vi "relay ladder.vi"() -> ()   [LabVIEW 2013]
panel:
  out "Array 2":bool[](array[boolean])
  in  "Knob 2":i32(knob) scale=0.0..250.0
  in  "stop 2":bool
  in  "Knob":i32(knob) scale=0.0..250.0
  in  "stop":bool
  out "Array":bool[](array[boolean])
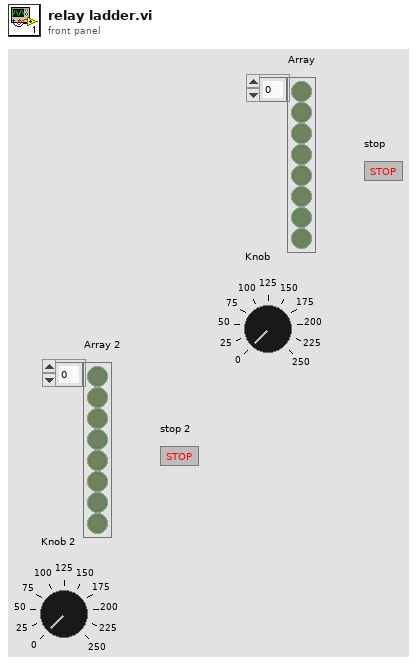
[diagram p1: front panel]
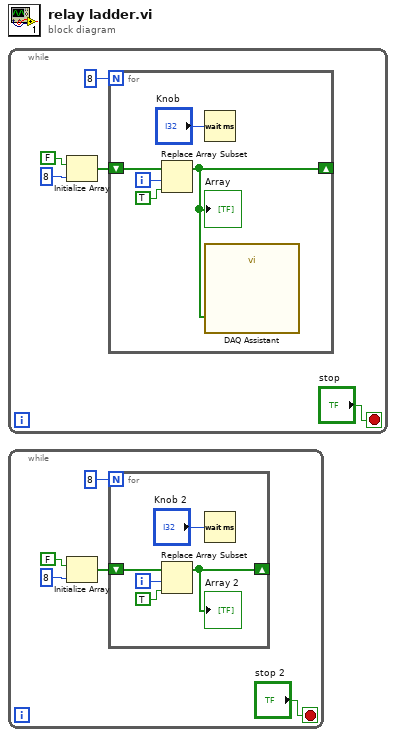
[diagram p0: block diagram]
diagram:
  n1 = while {
    stop <- "stop" stop-if-true
    n2 = Initialize Array(FALSE, 8 ("dimension size")) -> (w5:bool[])
    n3 = for {
      N: 8 -> [_]
      shift-right: [w7] -> _
      shift-left: w5 -> [w10]
      i -> [w9]
      n4 = Replace Array Subset(array=w10, new element=TRUE, index=w9) -> (w7:bool[])
      "Array" <- w7
      n5 = Wait (ms)(milliseconds to wait="Knob") -> ()  [unwired: 1 out]
      n6 = call "DAQ Assistant"("data"=w7) -> ()  [unwired: 17 in, 2 out]
    }
  }
  n7 = while {
    stop <- "stop 2" stop-if-true
    n8 = Initialize Array(FALSE, 8 ("dimension size")) -> (w15:bool[])
    n9 = for {
      N: 8 -> [_]
      shift-right: [w17] -> _
      shift-left: w15 -> [w20]
      i -> [w19]
      n10 = Replace Array Subset(array=w20, new element=TRUE, index=w19) -> (w17:bool[])
      "Array 2" <- w17
      n11 = Wait (ms)(milliseconds to wait="Knob 2") -> ()  [unwired: 1 out]
    }
  }
